vi "Remove Loose Ends.vi"(8 "error in (no error)":errorcluster, 11 "Assert VI Path":path) -> (0 "error out":errorcluster)   [LabVIEW 2018, in "Test.lvclass"]
doc: "Finds the main assert conditional disable structure in the assert vi and then deletes any loose ends left within it."
uses:
  Test.lvclass
  <vilib>/Utility/traverseref.llb/TRef TravTarget.ctl
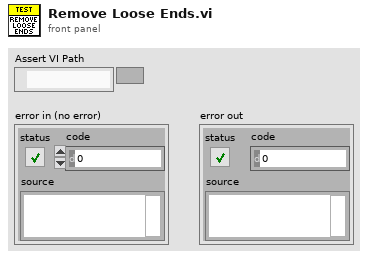
[diagram p1: front panel]
types:
  T1 = typedef "TRef TravTarget.ctl" = enum16{"FP", "BD", "Other"}
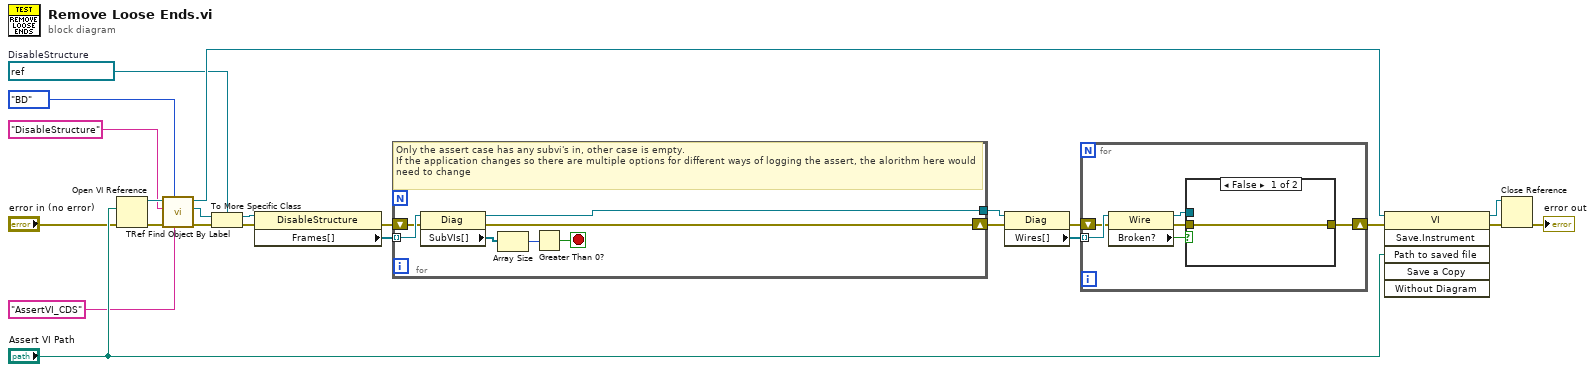
[diagram p0: block diagram]
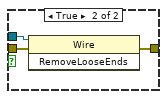
[diagram p2: hidden frame]
diagram:
  w11 = refnum<vi> refnum  # DisableStructure
  n1 = Open VI Reference(vi path="Assert VI Path", error in (no error)="error in (no error)") -> (vi reference=w18:refnum<vi>, error out=w14:errorcluster)  [unwired: 4 in]
  n2 = call <vilib>:"TRef Find Object By Label.vi"("Label"="AssertVI_CDS", "Traverse Target"=TRef_TravTarget."BD", "error in (no error)"=w14, "Class Name"="DisableStructure", "VI Ref"=w18) -> ("error out"=w12:errorcluster, "Found Obj Ref"=w13:refnum<vi>, "dup VI Ref"=w17:refnum<vi>)  [unwired: 3 in, 1 out]
  n3 = To More Specific Class(target class=w11, reference=w13, error in=w12) -> (specific class reference=w10:refnum<vi>, error out=w9:errorcluster)
  n4 = property class="DisableStructure"(reference=w10, error in=w9) -> (error out=w7:errorcluster, "Frames[]"=w8:refnum<vi>[])  [unwired: 1 out]
  n5 = for {
    tunnel: w8 -> [w30] mode=indexing
    shift-right: [w25] -> w5
    shift-left: w7 -> [w26]
    tunnel: [w24] -> w6
    stop <- w27 stop-if-true
    # "Only the assert case has any subvi's in, other case is empty.\nIf the application changes so there are multiple options for different ways of logging the assert, the alorithm here would need to change"
    n6 = property class="Diag"(reference=w30, error in=w26) -> (reference out=w24:refnum<vi>, error out=w25:errorcluster, "SubVIs[]"=w29:refnum<vi>[])
    n7 = Array Size(array=w29) -> (size(s)=w28:i32)
    n8 = Greater Than 0?(x=w28) -> (x > 0?=w27:bool)
  }
  n9 = property class="Diag"(reference=w6, error in=w5) -> (error out=w3:errorcluster, "Wires[]"=w4:refnum<vi>[])  [unwired: 1 out]
  n10 = for {
    tunnel: w4 -> [w36] mode=indexing
    shift-right: [w33] -> w2
    shift-left: w3 -> [w35]
    n11 = property class="Wire"(reference=w36, error in=w35) -> (reference out=w32:refnum<vi>, error out=w34:errorcluster, "Broken?"=w31:bool)
    n12 = case shown="False" w31 {
      tunnel: w34 -> [w37 w40]
      tunnel: [w37 w39] -> w33
      tunnel: w32 -> [_ w38]
      frame False {
      }
      frame True {
        n13 = invoke class="Wire" method="RemoveLooseEnds"(reference=w38, error in=w40) -> (error out=w39:errorcluster)  [unwired: 1 in, 2 out]
      }
    }
  }
  n14 = invoke class="VI" method="Save.Instrument"(reference=w17, error in=w2, "Path to saved file"="Assert VI Path") -> (reference out=w23:refnum<vi>, error out=w19:errorcluster)  [unwired: 3 in, 4 out]
  n15 = Close Reference(reference=w23, error in (no error)=w19) -> (error out=→"error out":errorcluster)
